vi "Cleanup.vi"(8 "error in (no error)":errorcluster, 11 "ControlArray in":refnum<class "ControlArray.lvclass">) -> (0 "error out":errorcluster)   [LabVIEW 2020, in "Control Array.lvlib" / "ControlArray.lvclass"]
uses:
  ControlArray.lvclass
  ControlArray.lvclass/ControlArray.ctl
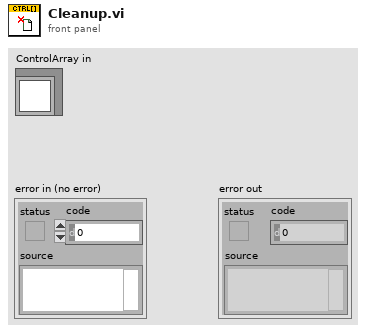
[diagram p1: front panel]
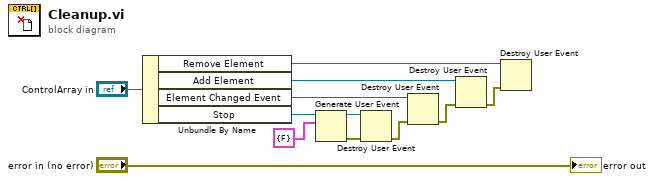
[diagram p0: block diagram]
diagram:
  n1 = Unbundle By Name("ControlArray in") -> ("Remove Element"=w2:refnum<user-event>, "Add Element"=w4:refnum<user-event>, "Element Changed Event"=w6:refnum<user-event>, "Stop"=w10:refnum<user-event>)
  n2 = Generate User Event(user event=w10, event data cluster=cluster{"Stop":bool} {"Stop"=FALSE} ("event data")) -> (user event out=w8:refnum<user-event>, error out=w7:errorcluster)  [unwired: 2 in]
  n3 = Destroy User Event(user event=w8, error in=w7) -> (error out=w5:errorcluster)
  n4 = Destroy User Event(user event=w6, error in=w5) -> (error out=w3:errorcluster)
  n5 = Destroy User Event(user event=w4, error in=w3) -> (error out=w1:errorcluster)
  n6 = Destroy User Event(user event=w2, error in=w1) -> ()  [unwired: 1 out]
  "error out" <- "error in (no error)"
